vi "UpdateInstance.vi"(8 "error in (no error)":errorcluster, 10 ".NET Refnum":refnum<k24>, 11 "Process in":refnum<class "Process.lvclass">) -> (0 "error out":errorcluster, 3 "Process out":refnum<class "Process.lvclass">)   [LabVIEW 2017, in "Process.lvclass"]
uses:
  Process.lvclass
  DLL/Modbus.dll
  Process.lvclass/Process.ctl
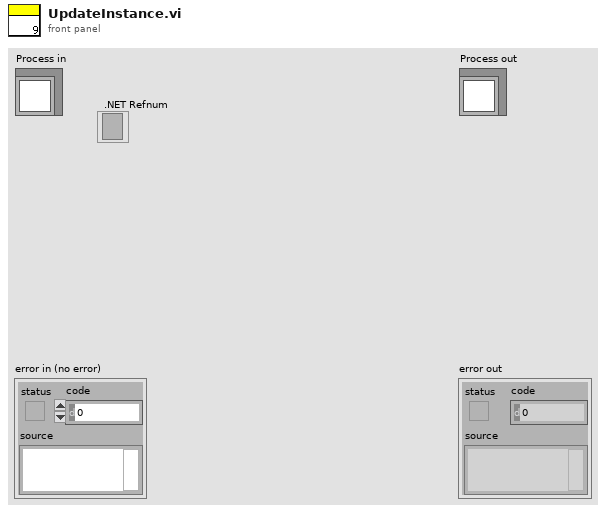
[diagram p1: front panel]
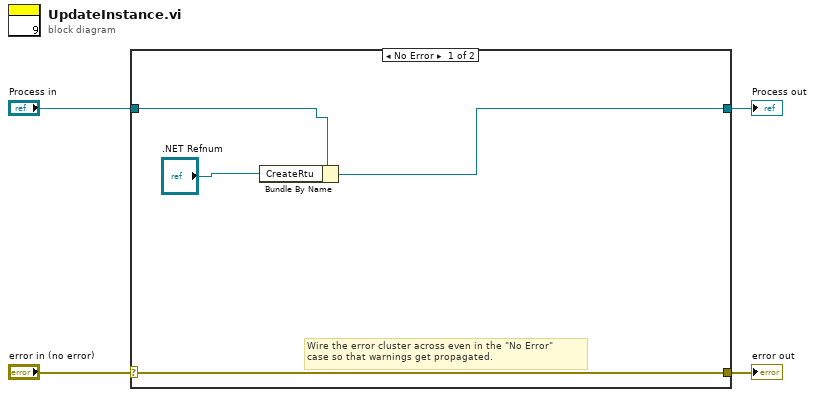
[diagram p0: block diagram]
diagram:
  n1 = case shown="No Error" "error in (no error)" {
    selector: "error in (no error)" -> [w8 w10]
    tunnel: [w8 w10] -> w3
    tunnel: [w6 w9] -> w1
    tunnel: "Process in" -> [w7 w9]
    frame No Error {
      # "Wire the error cluster across even in the \"No Error\"\ncase so that warnings get propagated."
      n2 = Bundle By Name(cluster=w7, "CreateRtu"=".NET Refnum") -> (w6:refnum<class "Process.lvclass">)
    }
    frame Error {
    }
  }
  "error out" <- w3
  "Process out" <- w1
